vi "Connect.vi"(8 "error in (no error)":errorcluster, 10 "Password":string, 11 "ByteGSWebAPI-V0 in":refnum<class "ByteGSWebAPI-V0.lvclass">) -> (0 "error out":errorcluster, 3 "ByteGSWebAPI-V0 out":refnum<class "ByteGSWebAPI-V0.lvclass">)   [LabVIEW 2019, in "ByteGSWebAPI.lvlib" / "ByteGSWebAPI-V0.lvclass"]
doc: "Effettua la connessione al server e richiede il token di accesso.\nIn caso in cui la connessione non avvenga o il token non venga restituito (password o user errati), restituisce un errore."
uses:
  ByteGSWebAPI-V0.lvclass
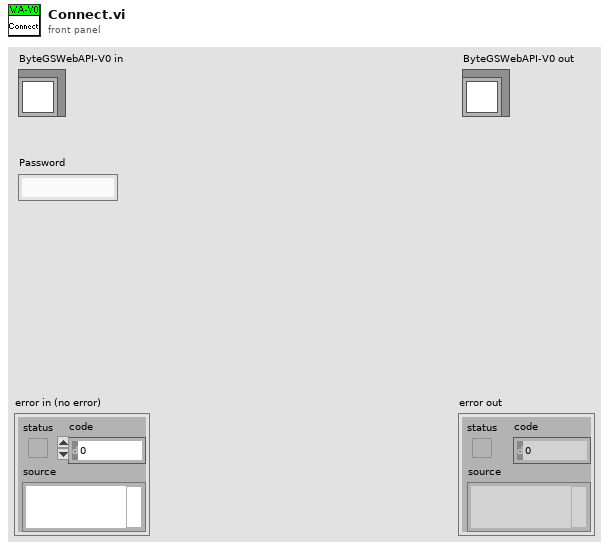
[diagram p1: front panel]
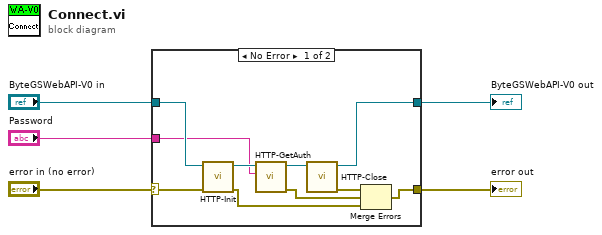
[diagram p0: block diagram]
diagram:
  n1 = case shown="No Error" "error in (no error)" {
    selector: "error in (no error)" -> [w9 w17]
    tunnel: [w8 w17] -> w4
    tunnel: [w10 w16] -> w2
    tunnel: "ByteGSWebAPI-V0 in" -> [w15 w16]
    tunnel: "Password" -> [w13 _]
    frame No Error {
      n2 = call "HTTP-Init.vi"("error in (no error)"=w9, "ByteGSWebAPI-V0 in"=w15) -> ("error out"=w6:errorcluster, "ByteGSWebAPI-V0 out"=w14:refnum<class "ByteGSWebAPI-V0.lvclass">)  [unwired: 8 in]
      n3 = call "HTTP-GetAuth.vi"("Password"=w13, "ByteGSWebAPI-V0 in"=w14) -> ("error out"=w7:errorcluster, "ByteGSWebAPI-V0 out"=w12:refnum<class "ByteGSWebAPI-V0.lvclass">)  [unwired: 8 in]
      n4 = call "HTTP-Close.vi"("ByteGSWebAPI-V0 in"=w12) -> ("error out"=w11:errorcluster, "ByteGSWebAPI-V0 out"=w10:refnum<class "ByteGSWebAPI-V0.lvclass">)  [unwired: 9 in]
      n5 = Merge Errors(w11, w7, w6) -> (w8:errorcluster)
    }
    frame Error {
    }
  }
  "error out" <- w4
  "ByteGSWebAPI-V0 out" <- w2
